vi "Axopatch_200B_ADC_config.vi"() -> (0 "DAC Outputs":tag[](array[tag]), 1 "DAC Inputs":tag[](array[tag]))   [LabVIEW 2014]
panel:
  in  "Mode":tag="DAC/ai3"
  in  "External Command Input":tag="DAC/ao0"
  in  "Gain":tag="DAC/ai2"
  in  "Output":tag="DAC/ai1"
  in  "Scaled Output":tag="DAC/ai0"
  # "Set connections with AXOPATCH 200B and DAQ card"
  # "INPUTS"
  # "I: alpha*beta mV/pA or V_m: aplha mV/mV"
  # "10 mV"
  # "alpha"
  # "OUTPUTS"
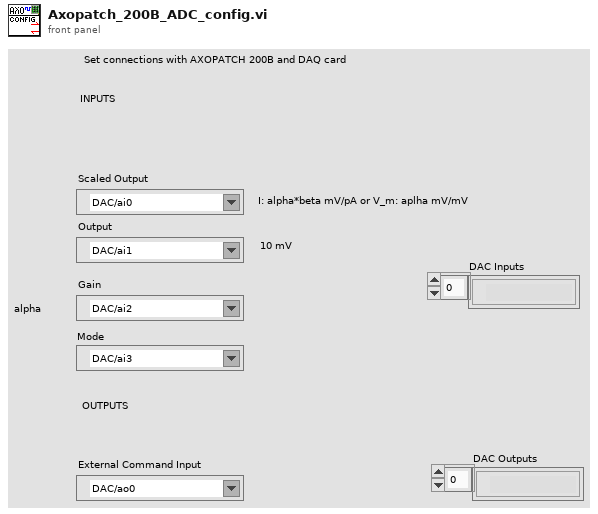
[diagram p1: front panel]
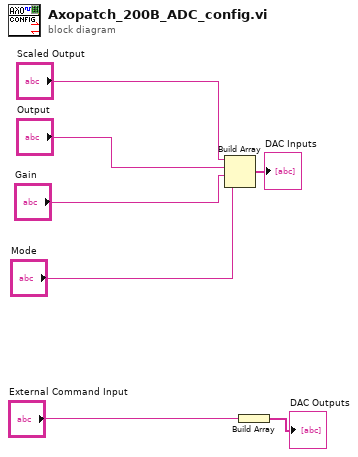
[diagram p0: block diagram]
diagram:
  n1 = Build Array("Scaled Output", "Output", "Gain", "Mode") -> (→"DAC Inputs":tag[])
  n2 = Build Array("External Command Input") -> (→"DAC Outputs":tag[])
